vi "gxml_BldArrayAttr.vi"(3 "Dim Sizes":i32[](array[numeric])) -> (1 "Dim Attr String":string)   [LabVIEW 2011, in "Third Party VIs.lvlib" / "GXML.lvlib"]
uses:
  GXML.lvlib
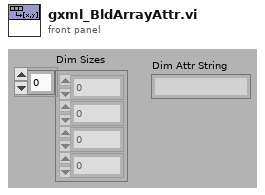
[diagram p1: front panel]
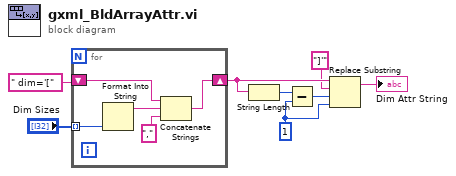
[diagram p0: block diagram]
diagram:
  w3 = 1 ("y")
  n1 = for {
    tunnel: "Dim Sizes" -> [w13] mode=indexing
    shift-right: [w9] -> w6
    shift-left: " dim='[" -> [w10]
    n2 = Format Into String(w13) -> (resulting string=w12:string)  [unwired: 3 in, 1 out]
    n3 = Concatenate Strings(w10, w12, "," ("string")) -> (w9:string)
  }
  n4 = String Length(string=w6) -> (length=w5:i32)
  n5 = Subtract(x=w5, y=w3) -> (x-y=w4:i32)
  n6 = Replace Substring(2:w3, 3:w4, 4:"]'", 5:w6) -> (1:→"Dim Attr String":string)  [unwired: 1 out]
